vi "索引数据并插入.vi"(8 "error in (no error)":errorcluster, 9 "数据类别":enum16{"水样数据", "日质控数据"}(ring), 10 "索引记录":timestamp format="%<%H:%M:%S\n%m/%d/%Y>T", 11 "table":string) -> (0 "error out":errorcluster, 3 "最新索引记录":timestamp)   [LabVIEW 2016, in "数据查询.lvlib"]
uses:
  <vilib>/addons/database/Connection.llb/DB Tools Open Connec (String).vi
  <vilib>/addons/database/_DB Variant To Data/Database Variant To Data.xnode
  <vilib>/addons/database/NI_Database_API.lvlib
panel:
  in  "data in":cluster{"时间":timestamp, "测量模式":string, "值":sgl}
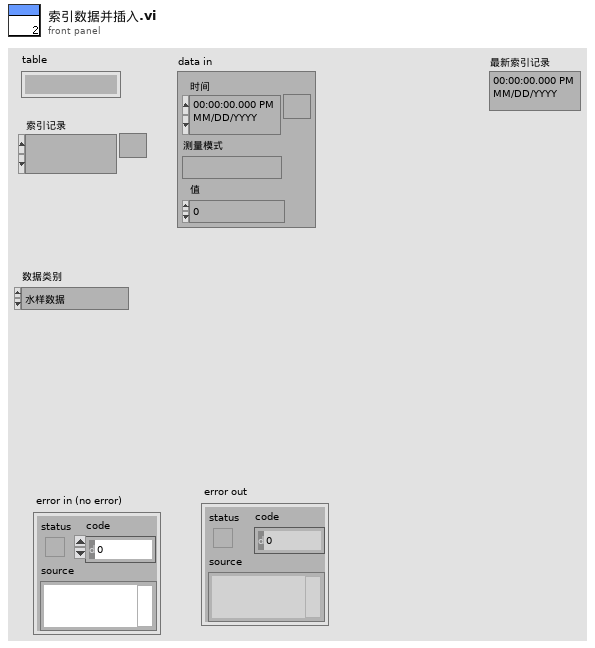
[diagram p1: front panel]
types:
  T1 = typedef "数据库类型.ctl" = enum16{"Access", "SQLite"}
  T2 = cluster{"时间":timestamp, "测量模式":string, "值":sgl}[]
  T3 = typedef "NI_Database_API.lvlib/Conn ObjectReference.ctl" = refnum<k1>
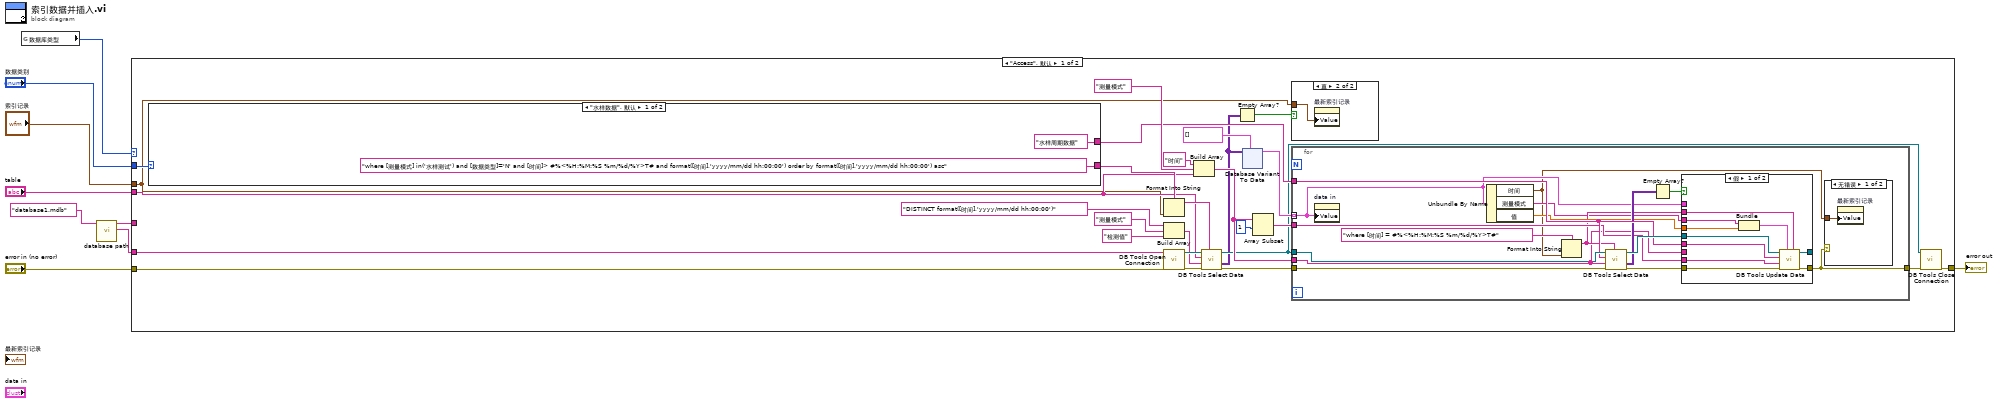
[diagram p0: block diagram]
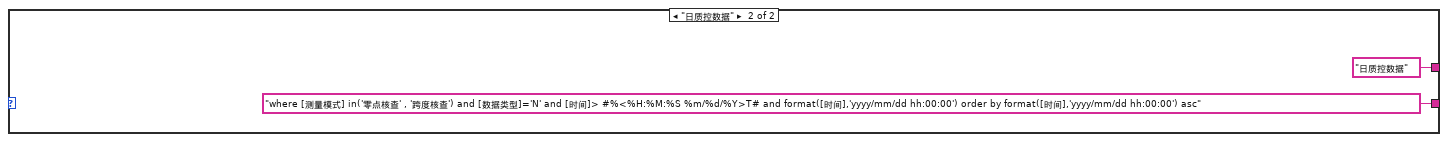
[diagram p3: hidden frame]
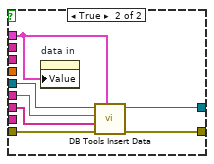
[diagram p5: hidden frame]
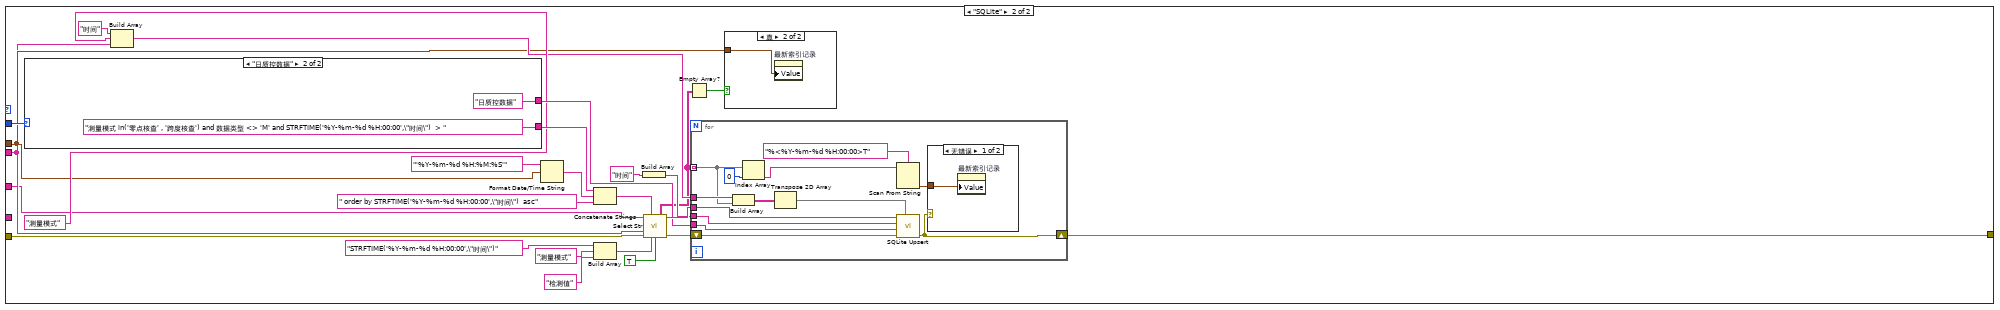
[diagram p6: hidden frame]
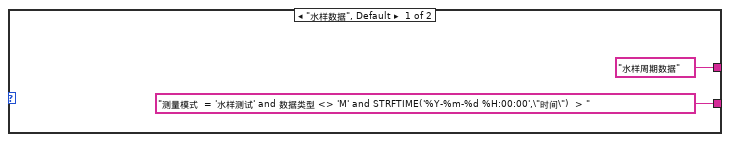
[diagram p9: hidden frame]
diagram:
  n1 = global read "外部调用接口全局变量.vi" "数据库类型"() -> (w1:T1)
  n2 = call "database path.vi"("database"="database1.mdb") -> ("Connection information"=w2:string, "Path out"=w3:string)  [unwired: 9 in]
  n3 = case shown="\"Access\", 默认" w1 {
    tunnel: "索引记录" -> [w12 w194]
    tunnel: "error in (no error)" -> [w27 w216]
    tunnel: [w26 w200] -> w5
    tunnel: "数据类别" -> [w20 w217]
    tunnel: "table" -> [w19 w193]
    tunnel: w3 -> [_ w192]
    tunnel: w2 -> [w10 _]
    frame "Access", Default {
      n4 = case shown="\"水样数据\", 默认" w20 {
        tunnel: ["where [测量模式] in('水样测试') and [数据类型]='N' and [时间]> #%<%H:%M:%S %m/%d/%Y>T# and format([时间],'yyyy/mm/dd hh:00:00') order by format([时间],'yyyy/mm/dd hh:00:00') asc" ("condition") "where [测量模式] in('零点核查' , '跨度核查') and [数据类型]='N' and [时间]> #%<%H:%M:%S %m/%d/%Y>T# and format([时间],'yyyy/mm/dd hh:00:00') order by format([时间],'yyyy/mm/dd hh:00:00') asc" ("condition")] -> w22
        tunnel: ["水样周期数据" "日质控数据"] -> w21
        frame "水样数据", Default {
        }
        frame "日质控数据" {
        }
      }
      n5 = Format Into String(format string=w22, w12) -> (resulting string=w32:string)  [unwired: 2 in, 1 out]
      n6 = Build Array("DISTINCT format([时间],'yyyy/mm/dd hh:00:00')", "测量模式" ("元素"), "检测值" ("元素")) -> (w31:string[])
      n7 = call-poly <vilib>:"DB Tools Open Connection.vi"("error in (no error)"=w27, "connection information"=w10) -> ("error out"=w33:errorcluster, "connection reference"=w34:T3)  [unwired: 6 in]
      n8 = Build Array("时间", "测量模式" ("元素"), w19) -> (w30:string[])
      n9 = call <vilib>:"DB Tools Select Data.vi"("condition"=w32, "error in (no error)"=w33, "columns"=w31, "table"=w19, "connection reference"=w34) -> ("error out"=w15:errorcluster, "data"=w13:variant[][], "connection reference out"=w16:T3)  [unwired: 1 in]
      n10 = Empty Array?(array=w13) -> (empty?=w11:bool)
      n11 = xnode "Database Variant To Data"("database variant"=w13, "type"=T2 []) -> ("data"=w17:T2)  [unwired: 1 in, 1 out]
      n12 = Array Subset(array=w30, index=1 ("索引")) -> (w28:string[])  [unwired: 1 in]
      n13 = case shown="真" w11 {
        tunnel: w12 -> [_ w37]
        frame False {
        }
        frame True {
          n14 = property on="最新索引记录" class="AbsTime (严格)"("Value"=w37) -> ()  [unwired: 2 in, 2 out]
        }
      }
      n15 = for {
        tunnel: w17 -> [w44] mode=indexing
        tunnel: w16 -> [w55]
        tunnel: w15 -> [w54]
        tunnel: [w43] -> w14
        tunnel: w21 -> [w51]
        tunnel: w30 -> [w46]
        tunnel: w28 -> [w48]
        n16 = property on="data in" class="Clust (严格)"("Value"=w44) -> ()  [unwired: 2 in, 2 out]
        n17 = Unbundle By Name(w44) -> ("时间"=w42:timestamp, "测量模式"=w45:string, "值"=w49:sgl)
        n18 = Format Into String(format string="where [时间] = #%<%H:%M:%S %m/%d/%Y>T#" ("condition"), w42) -> (resulting string=w47:string)  [unwired: 2 in, 1 out]
        n19 = call <vilib>:"DB Tools Select Data.vi"("condition"=w47, "error in (no error)"=w54, "columns"=w46, "table"=w51, "connection reference"=w55) -> ("error out"=w52:errorcluster, "data"=w50:variant[][], "connection reference out"=w53:T3)  [unwired: 1 in]
        n20 = Empty Array?(array=w50) -> (empty?=w56:bool)
        n21 = case shown="假" w56 {
          tunnel: w51 -> [w64 w75]
          tunnel: w53 -> [w68 w74]
          tunnel: w52 -> [w67 w73]
          tunnel: [w65 w71] -> w43
          tunnel: [w66 w72] -> _
          tunnel: w49 -> [w63 _]
          tunnel: w48 -> [w61 _]
          tunnel: w47 -> [w60 _]
          tunnel: w46 -> [_ w70]
          tunnel: w45 -> [w59 _]
          tunnel: w44 -> [_ w69]
          frame False {
            n22 = Bundle("测量模式"=w59, "值"=w63) -> (w62:cluster{"测量模式":string, "值":sgl})  [unwired: 1 in]
            n23 = call <vilib>:"DB Tools Update Data.vi"("condition"=w60, "data"=w62, "error in (no error)"=w67, "columns"=w61, "table"=w64, "connection reference"=w68) -> ("error out"=w65:errorcluster, "connection reference out"=w66:T3)  [unwired: 4 in]
          }
          frame True {
            n24 = property on="data in" class="Clust (严格)"("Value"=w69) -> ()  [unwired: 2 in, 2 out]
            n25 = call <vilib>:"DB Tools Insert Data.vi"("data"=w69, "error in (no error)"=w73, "columns"=w70, "table"=w75, "connection reference"=w74) -> ("error out"=w71:errorcluster, "connection reference out"=w72:T3)  [unwired: 5 in]
          }
        }
        n26 = case shown="无错误" w43 {
          tunnel: w42 -> [w58 _]
          frame No Error {
            n27 = property on="最新索引记录" class="AbsTime (严格)"("Value"=w58) -> ()  [unwired: 2 in, 2 out]
          }
          frame Error {
          }
        }
      }
      n28 = call <vilib>:"DB Tools Close Connection.vi"("error in (no error)"=w14, "connection reference"=w16) -> ("error out"=w26:errorcluster)  [unwired: 5 in]
    }
    frame "SQLite" {
      n29 = case shown="\"日质控数据\"" w217 {
        tunnel: ["测量模式  = '水样测试' and 数据类型 <> 'M' and STRFTIME('%Y-%m-%d %H:00:00',\"时间\")  > " ("condition") "测量模式 in('零点核查' , '跨度核查') and 数据类型 <> 'M' and STRFTIME('%Y-%m-%d %H:00:00',\"时间\")  > " ("condition")] -> w209
        tunnel: ["水样周期数据" "日质控数据"] -> w203
        frame "水样数据", Default {
        }
        frame "日质控数据" {
        }
      }
      n30 = Build Array("时间", "测量模式" ("元素"), w193) -> (w199:string[])
      n31 = Format Date/Time String(time format string (%c)="'%Y-%m-%d %H:%M:%S'" ("时间格式字符串(%c)"), seconds (now)=w194) -> (date/time string=w208:string)  [unwired: 1 in]
      n32 = Concatenate Strings(w209, w208, " order by STRFTIME('%Y-%m-%d %H:00:00',\"时间\")  asc" ("字符串")) -> (w206:string)
      n33 = Build Array("STRFTIME('%Y-%m-%d %H:00:00',\"时间\")", "测量模式" ("元素"), "检测值" ("元素")) -> (w212:string[])
      n34 = Build Array("时间") -> (w197:string[])
      n35 = call "Select Str.vi"("DB Path"=w192, "Where Clause"=w206, "Tables Name"=w193, "error in (no error)"=w216, "Columns"=w212, "Distinct"=TRUE) -> ("Results"=w196:string[][], "DB Path Out"=w204:string, "error out"=w205:errorcluster)  [unwired: 6 in, 1 out]
      n36 = Empty Array?(array=w196) -> (empty?=w195:bool)
      n37 = for {
        tunnel: w204 -> [w221]
        tunnel: w203 -> [w219]
        tunnel: w196 -> [w228] mode=indexing
        tunnel: w199 -> [w230]
        shift-right: [w223] -> w200
        shift-left: w205 -> [w231]
        tunnel: w197 -> [w220]
        n38 = Build Array(w230, w228) -> (w229:string[][])
        n39 = Index Array(array=w228, index=0 ("索引")) -> (element=w225:string)
        n40 = Transpose 2D Array(2D array=w229) -> (transposed array=w222:string[][])
        n41 = Scan From String(format string="%<%Y-%m-%d %H:00:00>T" ("格式字符串"), input string=w225) -> (output 1=w224:timestamp)  [unwired: 3 in, 3 out]
        n42 = call "SQLite Upsert.vi"("Column/Value Pairs"=w222, "错误输入（无错误）"=w231, "Table Name"=w219, "Constraint Columns"=w220, "DB Path"=w221) -> ("错误输出"=w223:errorcluster)  [unwired: 2 in, 2 out]
        n43 = case shown="无错误" w223 {
          tunnel: w224 -> [w232 _]
          frame No Error {
            n44 = property on="最新索引记录" class="AbsTime (严格)"("Value"=w232) -> ()  [unwired: 2 in, 2 out]
          }
          frame Error {
          }
        }
      }
      n45 = case shown="真" w195 {
        tunnel: w194 -> [_ w218]
        frame False {
        }
        frame True {
          n46 = property on="最新索引记录" class="AbsTime (严格)"("Value"=w218) -> ()  [unwired: 2 in, 2 out]
        }
      }
    }
  }
  "error out" <- w5
